vi "XML Reader Example.vi"(8 "error in":errorcluster, 11 "XML Path":path=path "C:/Users/tsanni/Desktop/Xml_test.xml") -> (0 "error out":errorcluster)   [LabVIEW 2016, in "Pathloss XML Reader.lvlib"]
uses:
  Pathloss XML Reader.lvlib
panel:
  out "Pathloss (dB)":dbl
  in  "Power":dbl format="%#_13g"
  in  "Frequency":dbl=3000000000.0 format="%#_13g"
  in  "Path Name":string="SignalPath"
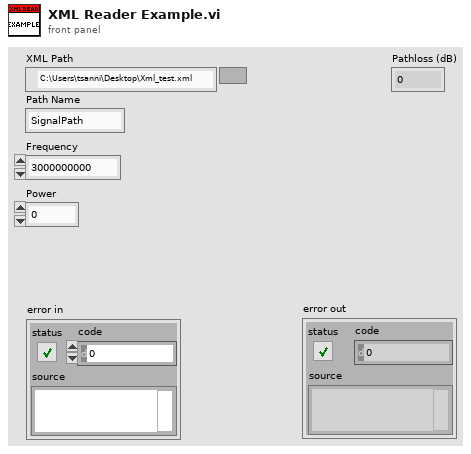
[diagram p1: front panel]
types:
  T1 = typedef "Pathloss XML Reader.lvlib/XML Reader Data Ref.ctl" = refnum<data-value>
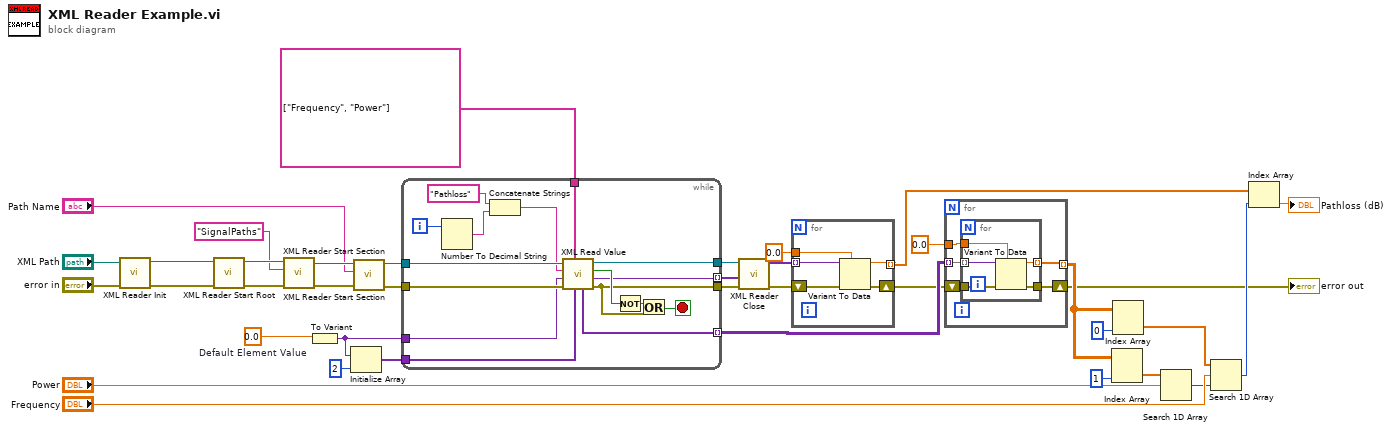
[diagram p0: block diagram]
diagram:
  w16 = 0.0  # Default Element Value
  n1 = call "XML Reader Init.vi"("error in"="error in", "File Path (dialog if empty)"="XML Path") -> ("error out"=w36:errorcluster, "XML Reader out"=w37:T1)  [unwired: 8 in]
  n2 = call "XML Reader Start Root.vi"("error in"=w36, "XML Reader In"=w37) -> ("error out"=w35:errorcluster, "XML Reader Out"=w34:T1)  [unwired: 8 in]
  n3 = call "XML Reader Start Section.vi"("error in"=w35, "Element Name"="SignalPaths" ("Section Name"), "XML Reader In"=w34) -> ("error out"=w33:errorcluster, "XML Reader Out"=w32:T1)  [unwired: 5 in, 2 out]
  n4 = To Variant(anything=w16) -> (Variant=w20:variant)
  n5 = Initialize Array(w20, 2 ("dimension size")) -> (w18:variant[])
  n6 = call "XML Reader Start Section.vi"("error in"=w33, "Element Name"="Path Name", "XML Reader In"=w32) -> ("error out"=w30:errorcluster, "XML Reader Out"=w31:T1)  [unwired: 5 in, 2 out]
  n7 = while {
    tunnel: w31 -> [w53]
    tunnel: w30 -> [w52]
    tunnel: [w44] -> w24
    tunnel: [w51] -> w29
    tunnel: w20 -> [w46]
    tunnel: [w42] -> w25 mode=indexing
    tunnel: string[] ["Frequency", "Power"] ("Attribute Names") -> [w40]
    tunnel: w18 -> [w39]
    tunnel: [w38] -> w17 mode=indexing
    i -> [w50]
    stop <- w43 stop-if-true
    n8 = Number To Decimal String(number=w50) -> (decimal integer string=w48:string)  [unwired: 1 in]
    n9 = Concatenate Strings("Pathloss" ("string"), w48) -> (w47:string)
    n10 = call "XML Read Value.vi"("Default Attribute Values"=w39, "Attribute Names"=w40, "error in (no error)"=w52, "Default Element Value"=w46, "Element Name"=w47, "XML Reader In"=w53) -> ("error out"=w44:errorcluster, "Element Value"=w42:variant, "Found?"=w45:bool, "XML Reader Out"=w51:T1, "Attribute Values"=w38:variant[])  [unwired: 1 in]
    n11 = Not(x=w45) -> (.not. x?=w41:bool)
    n12 = Or(x=w41, y=w44) -> (x .or. y?=w43:bool)
  }
  n13 = call "XML Reader Close.vi"("error in"=w24, "XML Reader In"=w29) -> ("error out"=w23:errorcluster)  [unwired: 9 in]
  n14 = for {
    tunnel: w25 -> [w58] mode=indexing
    tunnel: 0.0 ("Default Element Value") -> [w57]
    tunnel: [w55] -> w10 mode=indexing
    shift-right: [w54] -> w3
    shift-left: w23 -> [w56]
    n15 = Variant To Data(error in=w56, type=w57, Variant=w58) -> (data=w55:dbl, error out=w54:errorcluster)
  }
  n16 = for {
    tunnel: w17 -> [w63] mode=indexing
    tunnel: [w61] -> w7 mode=indexing
    shift-right: [w60] -> w1
    shift-left: w3 -> [w62]
    tunnel: 0.0 ("Default Element Value") -> [w59]
    n17 = for {
      tunnel: w63 -> [w68] mode=indexing
      tunnel: w62 -> [w67]
      tunnel: [w66] -> w61 mode=indexing
      tunnel: [w65] -> w60
      tunnel: w59 -> [w64]
      n18 = Variant To Data(error in=w67, type=w64, Variant=w68) -> (data=w66:dbl, error out=w65:errorcluster)
    }
  }
  "error out" <- w1
  n19 = Index Array(array=w7, index (col)=1 ("disabled index (col)")) -> (element=w13:dbl[])  [unwired: 1 in]
  n20 = Index Array(array=w7, index (col)=0 ("disabled index (col)")) -> (element=w6:dbl[])  [unwired: 1 in]
  n21 = Search 1D Array(1D array=w13, element="Power") -> (index of element=w11:i32)  [unwired: 1 in]
  n22 = Search 1D Array(1D array=w6, element="Frequency", start index (0)=w11) -> (index of element=w9:i32)
  n23 = Index Array(array=w10, index=w9) -> (element=→"Pathloss (dB)":dbl)
